vi "get start time tag.vi"() -> (3 "tag":refnum<class "tag descriptor.lvclass">)   [LabVIEW 2014, in "Shared Memory configuration.lvclass"]
uses:
  Shared Memory configuration.lvclass
  <vilib>/NI/Tag Bus/tag/tag descriptor.lvclass
  <vilib>/NI/Tag Bus/tag/Data Type.ctl
  <vilib>/NI/Tag Bus/tag/tag descriptor.lvclass/tag descriptor.ctl
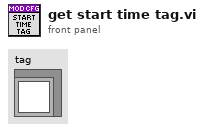
[diagram p1: front panel]
types:
  T1 = typedef "tag bus.lvlib/tag descriptor.lvclass/Data Type.ctl" = enum16{"Double", "Single", "I64", "I32", "I16", "I8", "U64", "U32", "U16", "U8", "Boolean", "String", "Array of Double", "Array of Single", "Array of I64", "Array of I32", "Array of I16", "Array of I8", "Array of U64", "Array of U32", "Array of U16", "Array of U8", "Array of Boolean", "Array of String"}
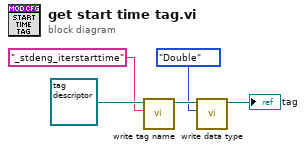
[diagram p0: block diagram]
diagram:
  n1 = call <vilib>:"write tag name.vi"("name"="_stdeng_iterstarttime" ("channel name"), "system tag in"=refnum<class "tag descriptor.lvclass"> refnum ("tag descriptor")) -> ("system tag out"=w4:refnum<class "tag descriptor.lvclass">)  [unwired: 8 in, 1 out]
  n2 = call <vilib>:"write data type.vi"("data type"=Data_Type."Double", "system tag in"=w4) -> ("system tag out"=→"tag":refnum<class "tag descriptor.lvclass">)  [unwired: 8 in, 1 out]
